vi "PWM_USART.vi"() -> ()   [LabVIEW 2021]
uses:
  <vilib>/Instr/_visa.llb/VISA Configure Serial Port (Instr).vi
panel:
  out "Waveform Chart":u8(graph)
  in  "DUTY":u8(slide) scale=0.0..100.0
  in  "flow control (0:none)":u16(ring) items=["None", "XON/XOFF", "RTS/CTS", "XON/XOFF & RTS/CTS", "DTR/DSR", "XON/XOFF & DTR/DSR"]
  in  "stop bits (10: 1 bit)":u16(ring)=10 items=["1.0"=10, "1.5"=15, "2.0"=20]
  in  "parity (0:none)":enum16{"None", "Odd", "Even", "Mark", "Space"}(ring)
  in  "data bits (8)":u16=8 min=5 max=8 step=1
  in  "baud rate (9600)":u32=9600
  in  "VISA resource name":refnum<visa-resource-name>
  in  "stop":bool
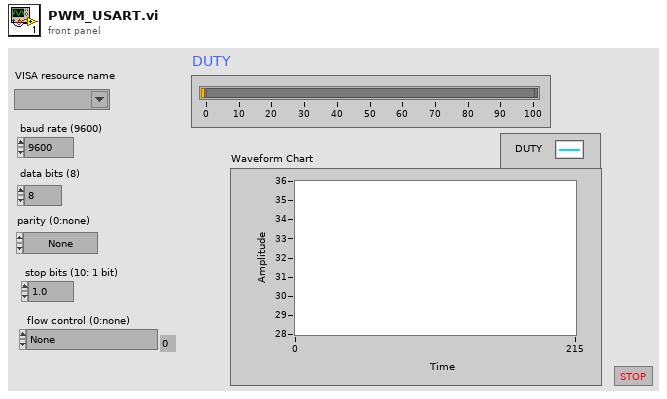
[diagram p1: front panel]
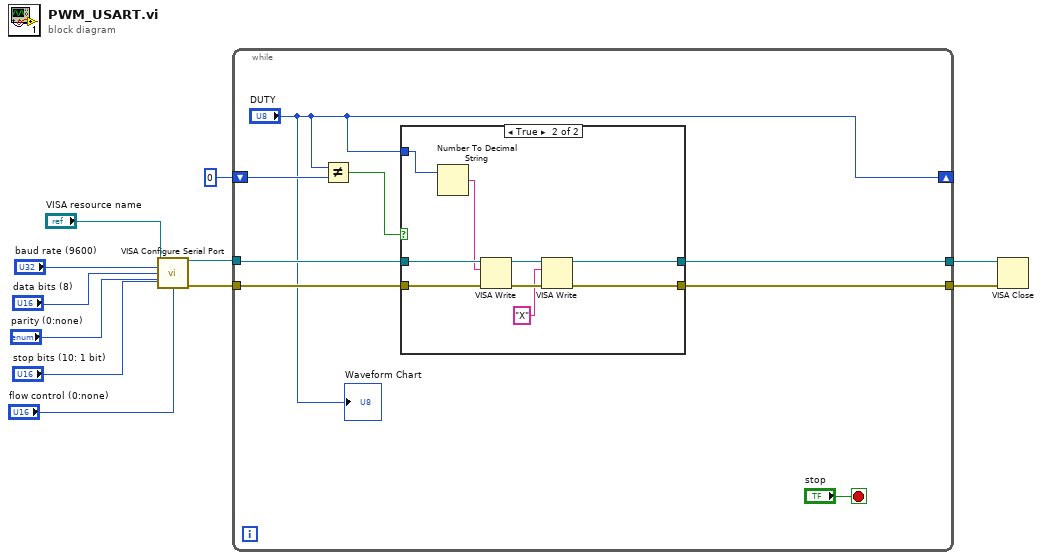
[diagram p0: block diagram]
diagram:
  n1 = call-poly "VISA Configure Serial Port"("VISA resource name"="VISA resource name", "baud rate (9600)"="baud rate (9600)", "data bits (8)"="data bits (8)", "parity (0:none)"="parity (0:none)", "stop bits (10: 1 bit)"="stop bits (10: 1 bit)", "flow control (0:none)"="flow control (0:none)") -> ("VISA resource name out"=w5:refnum<visa-resource-name>, "error out"=w4:errorcluster)  [unwired: 8 in]
  n2 = while {
    tunnel: w5 -> [w16]
    tunnel: w4 -> [w15]
    shift-right: ["DUTY"] -> _
    shift-left: 0 -> [w18]
    tunnel: [w14] -> w1
    tunnel: [w13] -> w2
    stop <- "stop" stop-if-true
    n3 = Not Equal?(x="DUTY", y=w18) -> (x != y?=w17:bool)
    n4 = case shown="True" w17 {
      tunnel: w16 -> [w21 w28]
      tunnel: w15 -> [w20 w29]
      tunnel: "DUTY" -> [_ w30]
      tunnel: [w21 w23] -> w13
      tunnel: [w20 w22] -> w14
      frame False {
      }
      frame True {
        n5 = Number To Decimal String(number=w30) -> (decimal integer string=w27:string)  [unwired: 1 in]
        n6 = VISA Write(VISA resource name=w28, write buffer=w27, error in (no error)=w29) -> (VISA resource name out=w25:refnum<visa-resource-name>, error out=w26:errorcluster)  [unwired: 1 out]
        n7 = VISA Write(VISA resource name=w25, write buffer="X", error in (no error)=w26) -> (VISA resource name out=w23:refnum<visa-resource-name>, error out=w22:errorcluster)  [unwired: 1 out]
      }
    }
    "Waveform Chart" <- "DUTY"
  }
  n8 = VISA Close(VISA resource name=w2, error in (no error)=w1) -> ()  [unwired: 1 out]
